vi "Collect-simulated-image.vi"(6 "Images in":T1[](array[typedef]), 7 "Index":i32, 8 "error in (no error)":errorcluster, 9 "Trigger ok?":bool, 10 "Config. params. ref. in":refnum<data-value>, 11 "Acquis. params. ref. in":refnum<data-value>) -> (0 "error out":errorcluster, 1 "Image ok?":bool, 2 "Config. params. ref.":refnum<data-value>, 3 "Acquis. params. ref.":refnum<data-value>, 4 "Images":T1[](array[typedef]))   [LabVIEW 2013, in "CameraVision.lvlib" / "CV-Acquisition.lvclass"]
uses:
  CV-Acquisition.lvclass
  Configuration/CV-Configuration.lvclass
  <vilib>/vision/Image Controls.llb/IMAQ Image.ctl
  Configuration/CV-Configuration.lvclass/CV-Configuration.ctl
  CV-Acquisition.lvclass/CV-Acquisition.ctl
  Configuration/Read Number of cameras.vi
  Read Image paths.vi
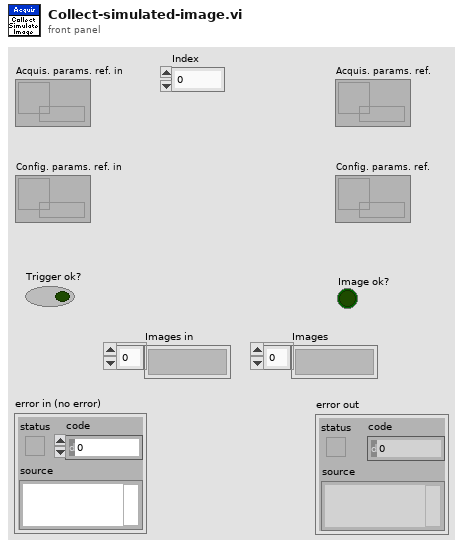
[diagram p1: front panel]
types:
  T1 = typedef "IMAQ Image.ctl" = refnum<image>
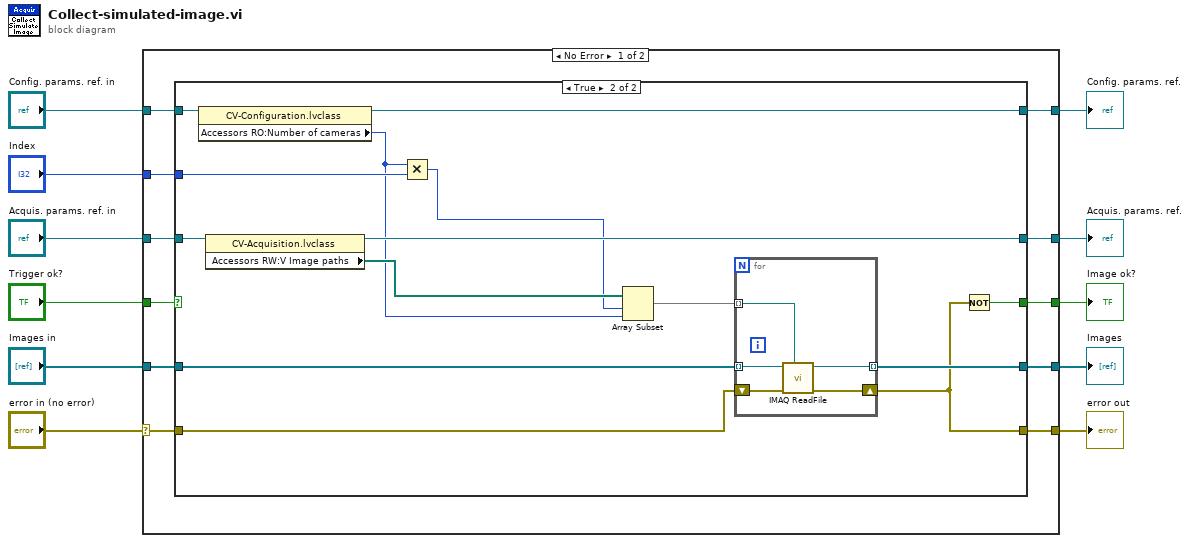
[diagram p0: block diagram]
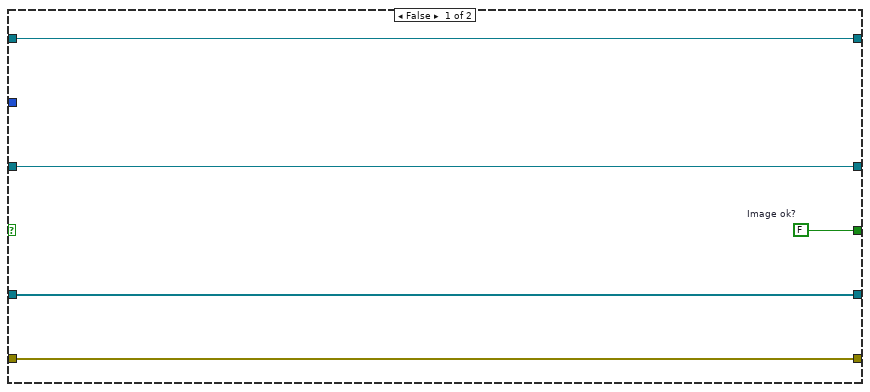
[diagram p2: hidden frame]
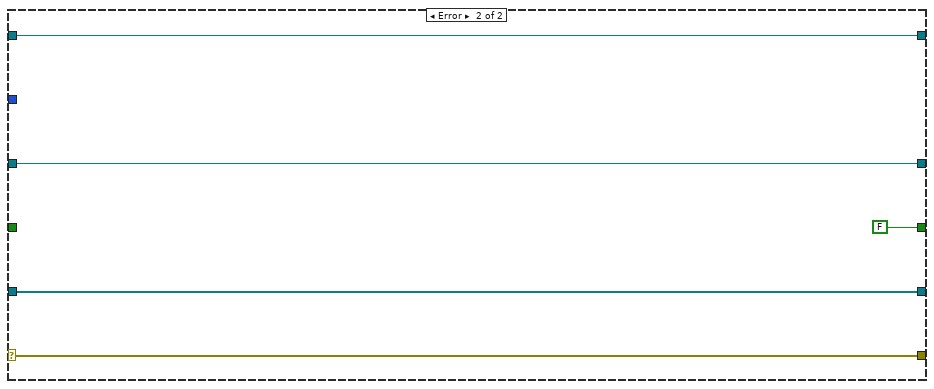
[diagram p3: hidden frame]
diagram:
  n1 = case shown="No Error" "error in (no error)" {
    selector: "error in (no error)" -> [w15 w51]
    tunnel: [w14 w51] -> w10
    tunnel: "Acquis. params. ref. in" -> [w22 w49]
    tunnel: [w13 w49] -> w6
    tunnel: [w20 w50] -> w7
    tunnel: "Config. params. ref. in" -> [w21 w50]
    tunnel: [w12 FALSE] -> w5
    tunnel: "Trigger ok?" -> [w19 _]
    tunnel: "Index" -> [w18 _]
    tunnel: "Images in" -> [w17 w47]
    tunnel: [w16 w47] -> w1
    frame No Error {
      n2 = case shown="True" w19 {
        tunnel: w22 -> [w25 w41]
        tunnel: w21 -> [w24 w40]
        tunnel: [w24 w39] -> w20
        tunnel: w18 -> [_ w38]
        tunnel: w17 -> [w27 w37]
        tunnel: [w27 w36] -> w16
        tunnel: w15 -> [w26 w35]
        tunnel: [w26 w28] -> w14
        tunnel: [w25 w34] -> w13
        tunnel: [w23 w29] -> w12
        frame False {
          w23 = FALSE  # Image ok?
        }
        frame True {
          n3 = property class="CV-Configuration.lvclass"(reference=w40) -> (reference out=w39:refnum<data-value>, "Accessors RO:Number of cameras"=w30:i32)  [unwired: 1 in, 1 out]
          n4 = property class="CV-Acquisition.lvclass"(reference=w41) -> (reference out=w34:refnum<data-value>, "Accessors RW:V Image paths"=w32:path[])  [unwired: 1 in, 1 out]
          n5 = Multiply(x=w30, y=w38) -> (x*y=w31:i32)
          n6 = Array Subset(array=w32, index=w31, length=w30) -> (w33:path[])
          n7 = for {
            tunnel: w33 -> [w46] mode=indexing
            tunnel: w37 -> [w45] mode=indexing
            tunnel: [w44] -> w36 mode=indexing
            shift-right: [w42] -> w28
            shift-left: w35 -> [w43]
            n8 = call "IMAQ ReadFile"("File Path"=w46, "error in (no error)"=w43, "Image"=w45) -> ("error out"=w42:errorcluster, "Image Out"=w44:T1)  [unwired: 4 in, 3 out]
          }
          n9 = Not(x=w28) -> (.not. x?=w29:bool)
        }
      }
    }
    frame Error {
    }
  }
  "error out" <- w10
  "Acquis. params. ref." <- w6
  "Config. params. ref." <- w7
  "Image ok?" <- w5
  "Images" <- w1
